vi "find_rects.vi"(5 "shrinkFactor":i32=1, 6 "Field of View":cluster{"fieldOfViewX":sgl, "fieldOfViewY":sgl}, 7 "logFileDir":string, 8 "error in":errorcluster, 9 "debug":bool, 10 "find_patches parameters":T2, 11 "Image":T3) -> (0 "error out":errorcluster, 2 "rects":T1(array[cluster]))   [LabVIEW 2017, in "gVision.lvlib"]
uses:
  gVision.lvlib
  <vilib>/vision/Image Controls.llb/IMAQ Image.ctl
  find_rects_parameters.ctl
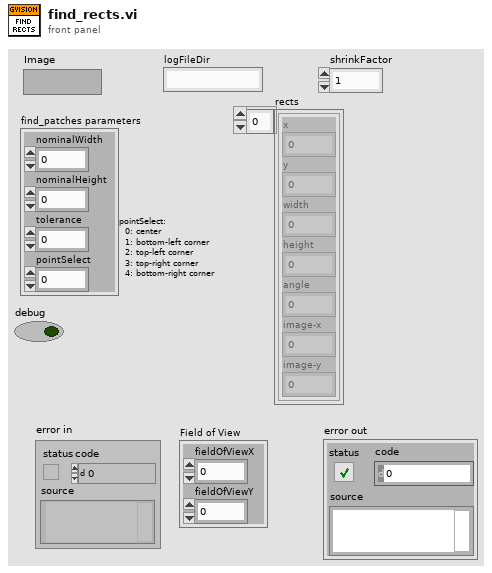
[diagram p1: front panel]
types:
  T1 = cluster{"x":dbl, "y":dbl, "width":dbl, "height":dbl, "angle":dbl, "image-x":dbl, "image-y":dbl}[]
  T2 = typedef "find_rects_parameters.ctl" = cluster{"nominalWidth":sgl, "nominalHeight":sgl, "tolerance":sgl, "pointSelect":sgl}
  T3 = typedef "IMAQ Image.ctl" = refnum<image>
  T4 = enum32{"Map Pixel Pointer", "Unmap Pixel Pointer", "Get Pixels Infos"}
  T5 = cluster{"x":dbl, "y":dbl, "width":dbl, "height":dbl, "angle":dbl, "image-x":dbl, "image-y":dbl}
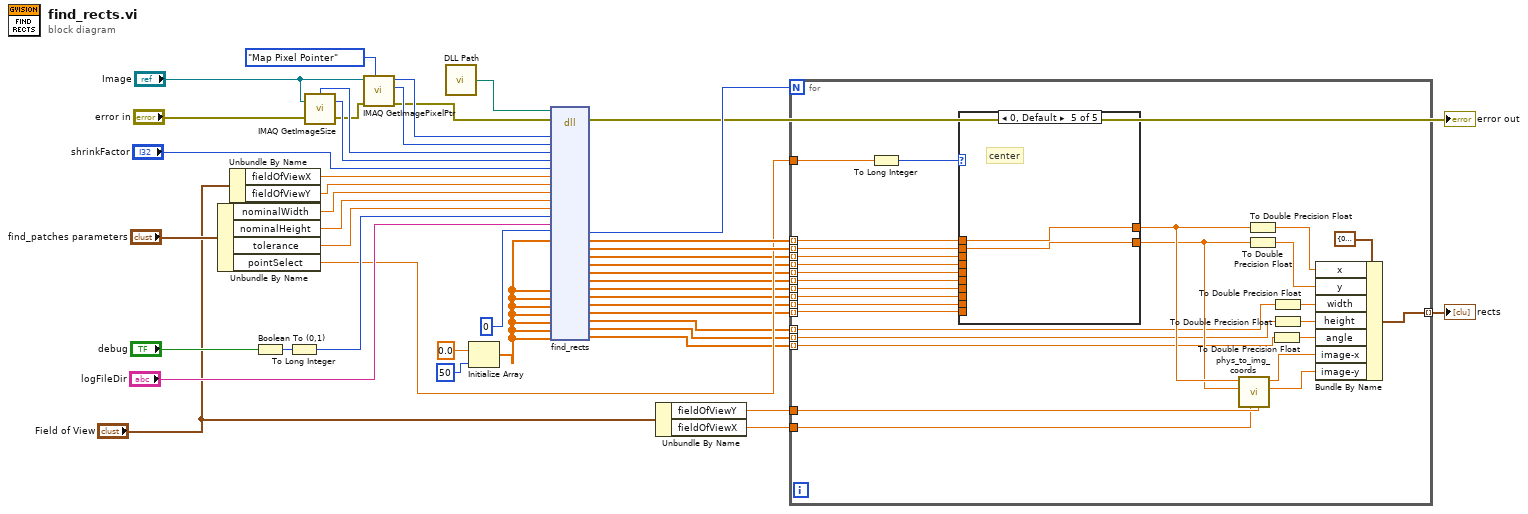
[diagram p0: block diagram]
diagram:
  n1 = Unbundle By Name("find_patches parameters") -> ("nominalWidth"=w28:sgl, "nominalHeight"=w27:sgl, "tolerance"=w26:sgl, "pointSelect"=w13:sgl)
  n2 = Unbundle By Name("Field of View") -> ("fieldOfViewX"=w31:sgl, "fieldOfViewY"=w30:sgl)
  n3 = Boolean To (0,1)(Boolean="debug") -> (0, 1=w24:i16)
  n4 = To Long Integer(number=w24) -> (32bit integer=w23:i32)
  n5 = call "IMAQ GetImageSize"("Image"="Image", "error in (no error)"="error in") -> ("Y Resolution"=w40:i32, "X Resolution"=w41:i32, "error out"=w34:errorcluster)  [unwired: 2 in]
  n6 = call "IMAQ GetImagePixelPtr"("Function"=T4."Map Pixel Pointer", "error in (no error)"=w34, "Image"="Image") -> ("error out"=w33:errorcluster, "LineWidth(Pixels)"=w42:i32, "Pixel Pointer out"=w43:u64)  [unwired: 3 in, 3 out]
  n7 = call "DLL Path.vi"() -> ("DLL Path"=w45:path)  [unwired: 5 in]
  n8 = Initialize Array(sgl 0.0 ("element"), 50 ("dimension size")) -> (w12:sgl[])
  n9 = dll-call lib="?" fn="find_rects"(path in=w45, error in=w33, "imgPtr"=w43, "imgLineWidth"=w42, "imgWidth"=w41, "imgHeight"=w40, "shrinkFactor"="shrinkFactor", "fieldOfViewX"=w31, "fieldOfViewY"=w30, "nominalWidth"=w28, "nominalHeight"=w27, "tolerance"=w26, "debug"=w23, "logFileDir"="logFileDir", "Nrects"=0, "rectXCenters"=w12, "rectYCenters"=w12, "rectXBLCorners"=w12, "rectYBLCorners"=w12, "rectXTLCorners"=w12, "rectYTLCorners"=w12, "rectXTRCorners"=w12, "rectYTRCorners"=w12, "rectXBRCorners"=w12, "rectYBRCorners"=w12, "rectWidths"=w12, "rectHeights"=w12, "rectAngles"=w12) -> (error out=→"error out":errorcluster, "Nrects"=w18:i32, "rectXCenters"=w17:sgl[], "rectYCenters"=w16:sgl[], "rectXBLCorners"=w8:sgl[], "rectYBLCorners"=w7:sgl[], "rectXTLCorners"=w6:sgl[], "rectYTLCorners"=w5:sgl[], "rectXTRCorners"=w4:sgl[], "rectYTRCorners"=w3:sgl[], "rectXBRCorners"=w2:sgl[], "rectYBRCorners"=w1:sgl[], "rectWidths"=w9:sgl[], "rectHeights"=w10:sgl[], "rectAngles"=w11:sgl[])  [unwired: 14 in, 1 out]
  n10 = Unbundle By Name("Field of View") -> ("fieldOfViewY"=w21:sgl, "fieldOfViewX"=w20:sgl)
  n11 = for {
    N: w18 -> [_]
    tunnel: w17 -> [w64] mode=indexing
    tunnel: w16 -> [w63] mode=indexing
    tunnel: [w73] -> w14 mode=indexing
    tunnel: w21 -> [w60]
    tunnel: w20 -> [w59]
    tunnel: w10 -> [w56] mode=indexing
    tunnel: w13 -> [w57]
    tunnel: w11 -> [w55] mode=indexing
    tunnel: w9 -> [w54] mode=indexing
    tunnel: w8 -> [w53] mode=indexing
    tunnel: w7 -> [w52] mode=indexing
    tunnel: w6 -> [w51] mode=indexing
    tunnel: w5 -> [w50] mode=indexing
    tunnel: w4 -> [w49] mode=indexing
    tunnel: w3 -> [w48] mode=indexing
    tunnel: w2 -> [w47] mode=indexing
    tunnel: w1 -> [w46] mode=indexing
    n12 = To Long Integer(number=w57) -> (32bit integer=w58:i32)
    n13 = case shown="0, Default" w58 {
      tunnel: w64 -> [_ _ _ _ w83]
      tunnel: w63 -> [_ _ _ _ w82]
      tunnel: [w75 w77 w79 w81 w83] -> w62
      tunnel: [w74 w76 w78 w80 w82] -> w61
      tunnel: w53 -> [w75 _ _ _ _]
      tunnel: w52 -> [w74 _ _ _ _]
      tunnel: w51 -> [_ w77 _ _ _]
      tunnel: w50 -> [_ w76 _ _ _]
      tunnel: w49 -> [_ _ w79 _ _]
      tunnel: w48 -> [_ _ w78 _ _]
      tunnel: w47 -> [_ _ _ w81 _]
      tunnel: w46 -> [_ _ _ w80 _]
      frame 1 {
        # "bottom-left"
      }
      frame 2 {
        # "top-left"
      }
      frame 3 {
        # "top-right"
      }
      frame 4 {
        # "bottom-right"
      }
      frame 0, Default {
        # "center"
      }
    }
    n14 = call "phys_to_img_coords.vi"("fov_y"=w60, "fov_x"=w59, "y"=w61, "x"=w62) -> ("image_y"=w68:dbl, "image_x"=w69:dbl)  [unwired: 6 in]
    n15 = To Double Precision Float(number=w62) -> (double precision float=w72:dbl)
    n16 = To Double Precision Float(number=w61) -> (double precision float=w71:dbl)
    n17 = To Double Precision Float(number=w55) -> (double precision float=w65:dbl)
    n18 = To Double Precision Float(number=w54) -> (double precision float=w70:dbl)
    n19 = To Double Precision Float(number=w56) -> (double precision float=w67:dbl)
    n20 = Bundle By Name(cluster=T5 {"x"=0.0, "y"=0.0, "width"=0.0, "height"=0.0, "angle"=0.0, "image-x"=0.0, "image-y"=0.0}, "x"=w72, "y"=w71, "width"=w70, "height"=w67, "angle"=w65, "image-x"=w69, "image-y"=w68) -> (w73:T5)
  }
  "rects" <- w14
